vi "ISOSPI_DELTAVCELL.vi"(8 "errin":errorcluster, 9 "nbmodule":i32=8, 11 "visain":refnum<visa-resource-name>) -> (0 "errout":errorcluster, 2 "NTC Temperatures":string[][](table), 3 "Cell Voltages":string[][](table), 4 "TCellmax":dbl, 5 "VCellmax":dbl, 6 "TCellmin":dbl, 7 "VCellmin":dbl)   [LabVIEW 2020]
panel:
  out "deltaV":dbl[](array[numeric])
  out "Tension OUT":dbl[][](array[numeric])
  out "?":bool
  in  "stop":bool
  # "CMU ANALYSER"
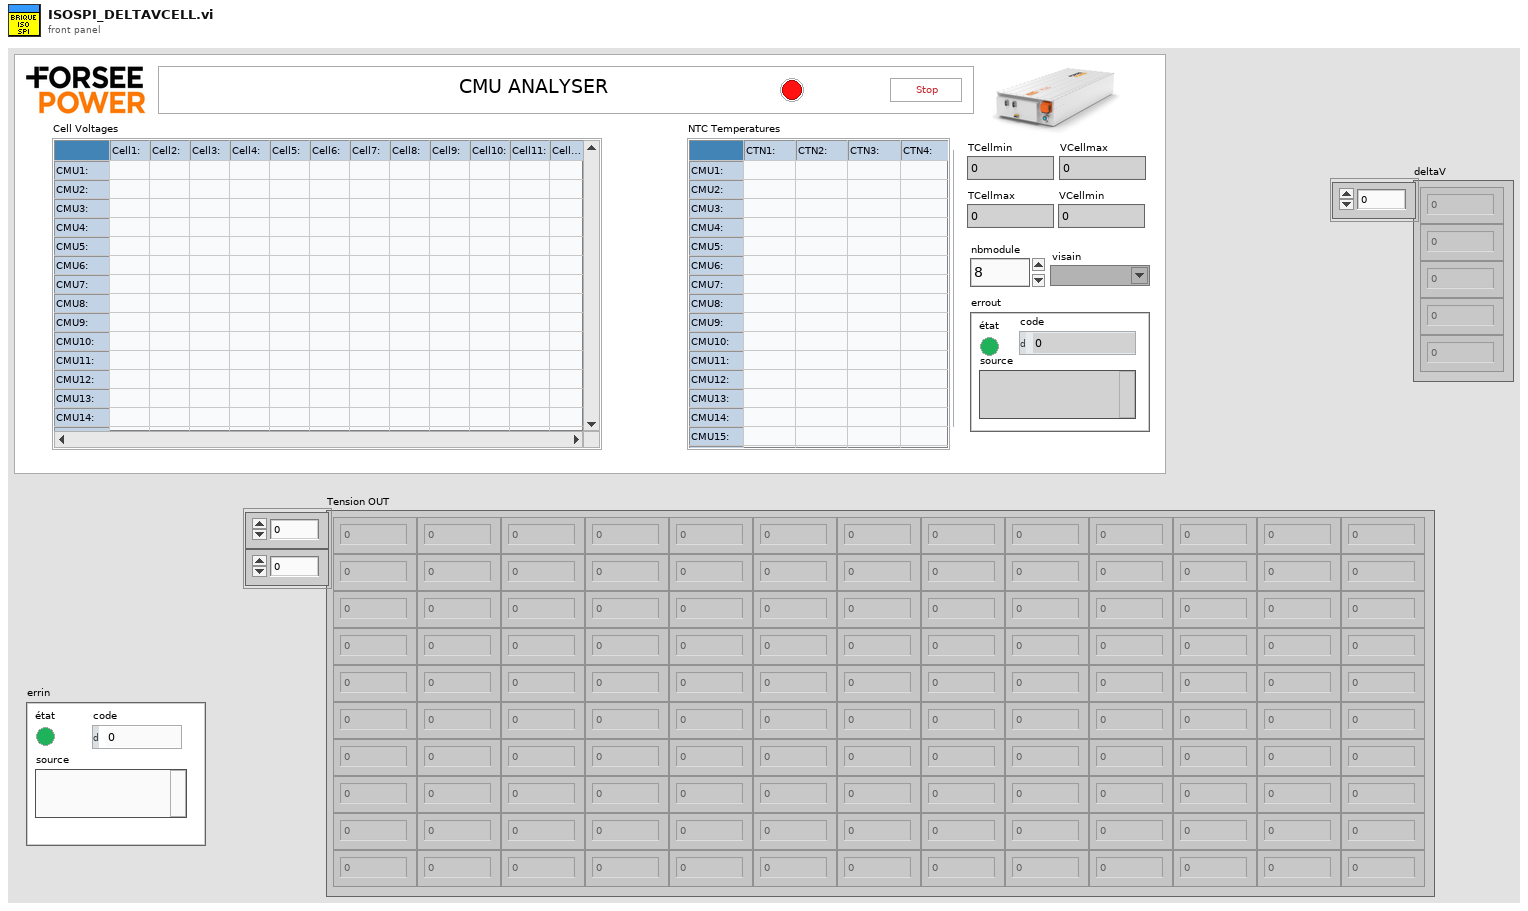
[diagram p1: front panel]
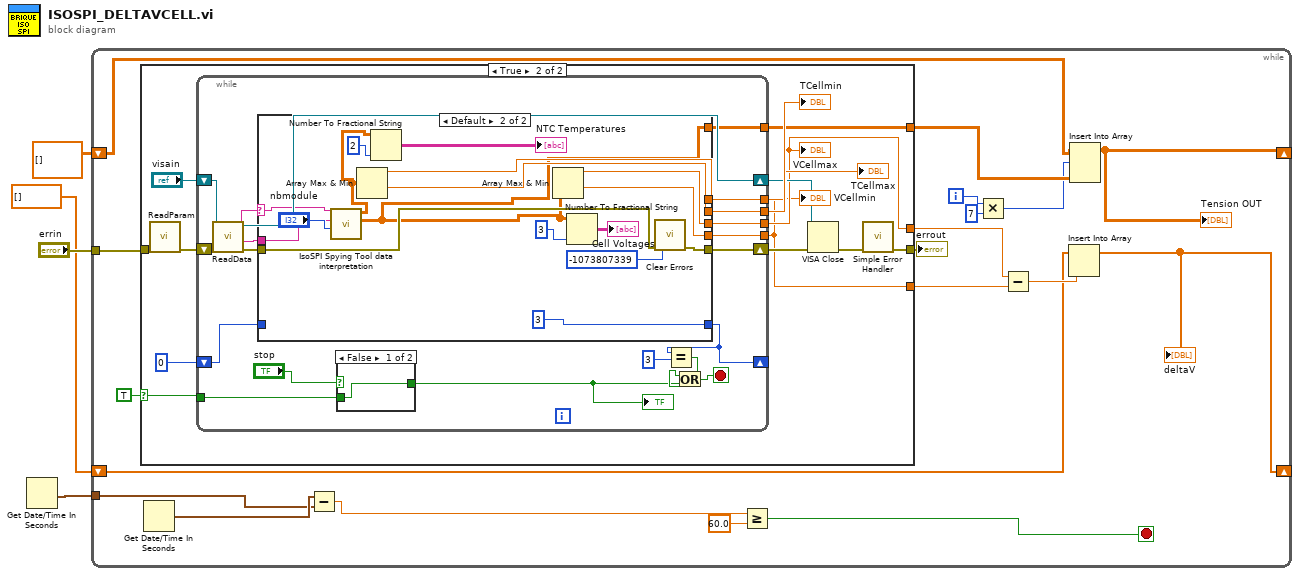
[diagram p0: block diagram]
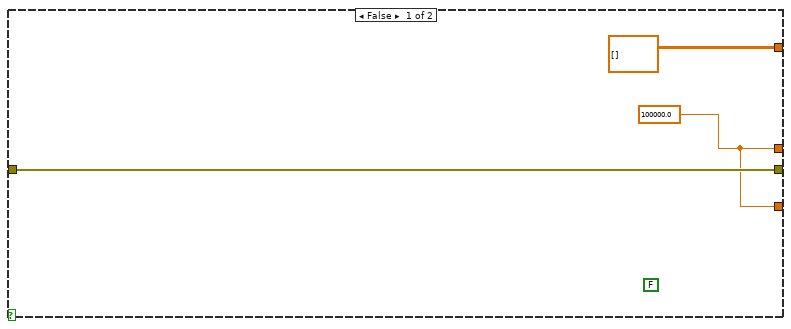
[diagram p2: hidden frame]
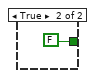
[diagram p3: hidden frame]
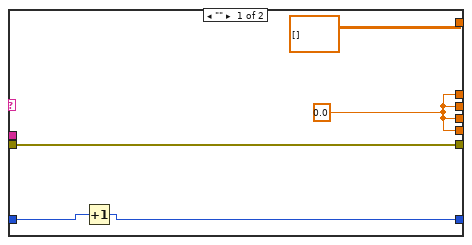
[diagram p4: hidden frame]
diagram:
  n1 = Get Date/Time In Seconds() -> (seconds since 1Jan1904=w3:timestamp)
  n2 = while {
    tunnel: "errin" -> [w22]
    tunnel: w3 -> [w10]
    shift-right: [w13] -> _
    shift-left: dbl[][] [] -> [w12]
    shift-right: [w5] -> _
    shift-left: dbl[] [] ("array") -> [w6]
    i -> [w16]
    stop <- w18 stop-if-true
    n3 = case shown="True" TRUE {
      selector: TRUE -> [_ w30]
      tunnel: [w26 w38] -> w23
      tunnel: w22 -> [w26 w37]
      tunnel: [dbl[][] [] ("TCELL") w29] -> w17
      tunnel: [w24 w28] -> w9
      tunnel: [w24 w27] -> w8
      frame False {
        w24 = 100000.0
        (unwired) FALSE
      }
      frame True {
        n4 = call "ReadParam.vi"("error in (no error)"=w37) -> ("error out"=w32:errorcluster)  [unwired: 10 in]
        n5 = while {
          shift-right: [w60] -> w35
          shift-left: "visain" -> [w59]
          shift-right: [w54] -> w36
          shift-left: w32 -> [w53]
          tunnel: [w58] -> w28
          tunnel: [w57] -> w27
          tunnel: [w56] -> w39
          tunnel: [w55] -> w40
          shift-right: [w49] -> _
          shift-left: 0 ("x") -> [w51]
          tunnel: w30 -> [w43]
          tunnel: [w41] -> w29
          stop <- w42 stop-if-true
          n6 = call "ReadData.vi"("errin"=w53, "visain"=w59) -> ("errout"=w52:errorcluster, "TResult"=w47:string, "VResult"=w48:string, "visaout"=w60:refnum<visa-resource-name>)  [unwired: 6 in]
          n7 = case shown="Default" w48 {
            selector: w48 -> [_ w71]
            tunnel: [w67 w84] -> w58
            tunnel: [w67 w83] -> w57
            tunnel: [w67 w82] -> w56
            tunnel: [w67 w81] -> w55
            tunnel: [w66 w77] -> w54
            tunnel: w52 -> [w66 w76]
            tunnel: w51 -> [w65 _]
            tunnel: [w64 3] -> w49
            tunnel: w47 -> [_ w72]
            tunnel: [dbl[][] [] ("TCELL") w68] -> w41
            frame "" {
              w67 = 0.0
              n8 = Increment(x=w65) -> (x+1=w64:i32)
            }
            frame Default {
              n9 = call "IsoSPI Spying Tool data interpretation.vi"("nbmodule"="nbmodule", "TCell"=w72, "VCell"=w71) -> ("Vcell"=w68:dbl[][], "TCELL"=w69:dbl[][])  [unwired: 7 in]
              n10 = Array Max & Min(array=w69) -> (max value=w82:dbl, min value=w81:dbl)  [unwired: 2 out]
              n11 = Number To Fractional String ("Nombre en chaîne fractionnaire")(number=w69, precision (6)=i16 2 ("précision (6)")) -> (F-format string=→"NTC Temperatures":string[][])  [unwired: 2 in]
              n12 = Array Max & Min(array=w68) -> (max value=w84:dbl, min value=w83:dbl)  [unwired: 2 out]
              n13 = Number To Fractional String ("Nombre en chaîne fractionnaire")(number=w68, precision (6)=i16 3 ("précision (6)")) -> (F-format string=→"Cell Voltages":string[][])  [unwired: 2 in]
              n14 = call <vilib>:"Clear Errors.vi"("error in (no error)"=w76, "specific error code to clear (0: all)"=-1073807339) -> ("error out"=w77:errorcluster)  [unwired: 4 in, 1 out]
            }
          }
          n15 = case shown="False" "stop" {
            tunnel: [w61 FALSE] -> w44
            tunnel: w43 -> [w61 _]
            frame False {
            }
            frame True {
            }
          }
          "?" <- w44
          n16 = Equal? ("Égaux ?")(x=w49, y=3) -> (x = y?=w46:bool)
          n17 = Or(x=w46, y=w44) -> (x .or. y?=w42:bool)
        }
        "TCellmin" <- w40
        "TCellmax" <- w39
        "VCellmin" <- w27
        "VCellmax" <- w28
        n18 = VISA Close(VISA resource name=w35, error in (no error)=w36) -> (error out=w34:errorcluster)
        n19 = call <vilib>:"Simple Error Handler.vi"("error in (no error)"=w34) -> ("error out"=w38:errorcluster)  [unwired: 4 in, 4 out]
      }
    }
    "errout" <- w23
    n20 = Get Date/Time In Seconds() -> (seconds since 1Jan1904=w11:timestamp)
    n21 = Subtract(x=w11, y=w10) -> (x-y=w20:dbl)
    n22 = Greater Or Equal?(x=w20, y=60.0) -> (x >= y?=w18:bool)
    n23 = Multiply(x=w16, y=7) -> (x*y=w14:i32)
    n24 = Subtract(x=w9, y=w8) -> (x-y=w7:dbl)
    n25 = Insert Into Array(array=w6, new element=w7) -> (w5:dbl[])  [unwired: 1 in]
    "deltaV" <- w5
    n26 = Insert Into Array(array=w12, index (row)=w14, new element=w17) -> (w13:dbl[][])  [unwired: 1 in]
    "Tension OUT" <- w13
  }
